vi "ATS_Prefix_to_Numeric.vi"(7 "String":string) -> (1 "10^Prefix":dbl format="%.2e", 2 "number":dbl format="%.2e", 3 "Full Value":dbl format="%.2e")   [LabVIEW 2014]
doc: "_____AlazarTech, Scope_____\n\nConvert the input String with prefix in Real number."
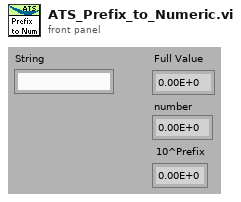
[diagram p1: front panel]
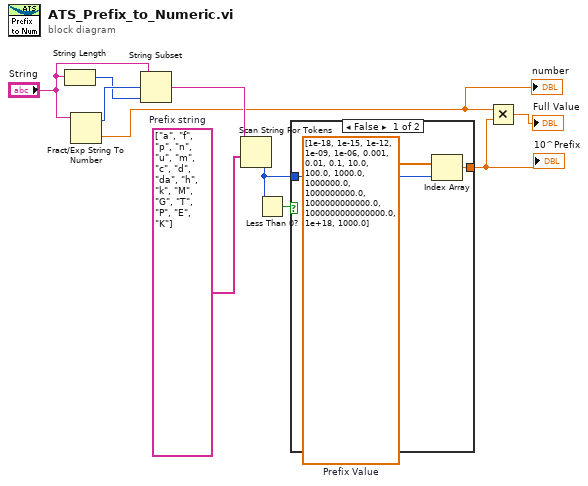
[diagram p0: block diagram]
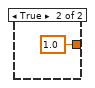
[diagram p2: hidden frame]
diagram:
  w10 = string[] ["a", "f", "p", "n", "u", "m", "c", "d", "da", "h", "k", "M", "G", "T", "P", "E", "K"]  # Prefix string
  n1 = String Length(string="String") -> (length=w2:i32)
  n2 = Fract/Exp String To Number(string="String") -> (offset past number=w3:i32, number=w5:dbl)  [unwired: 3 in]
  "number" <- w5
  n3 = String Subset(string="String", offset (0)=w3, length (rest)=w2) -> (substring=w7:string)
  n4 = Scan String For Tokens(7:w10, 9:w7) -> (0:w9:i32)  [unwired: 4 in, 3 out]
  n5 = Less Than 0?(x=w9) -> (x < 0?=w8:bool)
  n6 = case shown="False" w8 {
    tunnel: w9 -> [w12 _]
    tunnel: [w11 1.0] -> w6
    frame False {
      w13 = dbl[] [1e-18, 1e-15, 1e-12, 1e-09, 1e-06, 0.001, 0.01, 0.1, 10.0, 100.0, 1000.0, 1000000.0, 1000000000.0, 1000000000000.0, 1000000000000000.0, 1e+18, 1000.0]  # Prefix Value
      n7 = Index Array(array=w13, index=w12) -> (element=w11:dbl)
    }
    frame True {
    }
  }
  "10^Prefix" <- w6
  n8 = Multiply(x=w5, y=w6) -> (x*y=→"Full Value":dbl)
